vi "GetEdge.vi"(1 "Measurement Source (1: Channel 1)":i32(ring)=1 caption="Channel (1: Channel 1)" items=["Channel 1"=1, "Channel 2"=2, "Channel 3"=3, "Channel 4"=4, "Function 1"=5, "Function 2"=6, "Function 3"=7, "Function 4"=8, "Memory 1"=9, "Memory 2"=10, "Memory 3"=11, "Memory 4"=12, "Clock"=15, "MTrend"=16, "MSpectrum"=17, "Equalized"=18, "DIG 0"=20, "DIG 1"=21, "DIG 2"=22, "DIG 3"=23, "DIG 4"=24, "DIG 5"=25, "DIG 6"=26, "DIG 7"=27, "DIG 8"=28, "DIG 9"=29, "DIG 10"=30, "DIG 11"=31, "DIG 12"=32, "DIG 13"=33, "DIG 14"=34, "DIG 15"=35], 2 "VISA resource name":refnum<visa-resource-name>) -> (0 "Time Interval (s)":dbl)   [LabVIEW 2014]
uses:
  <instrlib>/Agilent 90000 Series/Public/Data/Read Measurement (Time Edge Interval).vi
  <instrlib>/Agilent 90000 Series/Agilent 90000 Series.lvlib
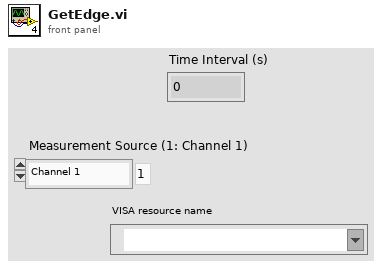
[diagram p1: front panel]
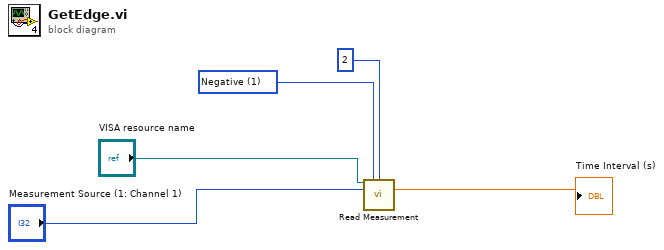
[diagram p0: block diagram]
diagram:
  w4 = 1 items=["Positive", "Negative"] ("Slope (0:Positive)")
  n1 = call-poly <instrlib>:"Read Measurement.vi"("VISA resource name"="VISA resource name", "Slope (0:Positive)"=w4, "Occurrence (3)"=2, "Measurement Source (1: Channel 1)"="Measurement Source (1: Channel 1)") -> ("Time Interval (s)"=→"Time Interval (s)":dbl)  [unwired: 9 in, 2 out]
